vi "Search Remote Session.vi"(8 "error in":errorcluster) -> (0 "error out":errorcluster, 1 "Errors per session try":string[](array[string]), 2 "sessions out":string[][](array[string]))   [LabVIEW 2024, in "Session Scanner.lvlib"]
uses:
  Session Scanner.lvlib
  <vilib>/net/SSH/Client/OpenSSH/OpenSSH Client.lvclass
  C:/Program Files (x86)/National Instruments/LabVIEW 2024/vi.lib/net/SSH/Client/Generic/Generic Client.lvclass
  <vilib>/net/SSH/Client/Generic/Generic Client.lvclass/Generic Client.ctl
  <vilib>/net/SSH/Client/Generic/Write trust on first use.vi
  Support/General Type Defs/Global Data.vi
  <vilib>/net/SSH/NI_SSH.lvlib
  Support/General Type Defs/General Type Defs.lvlib
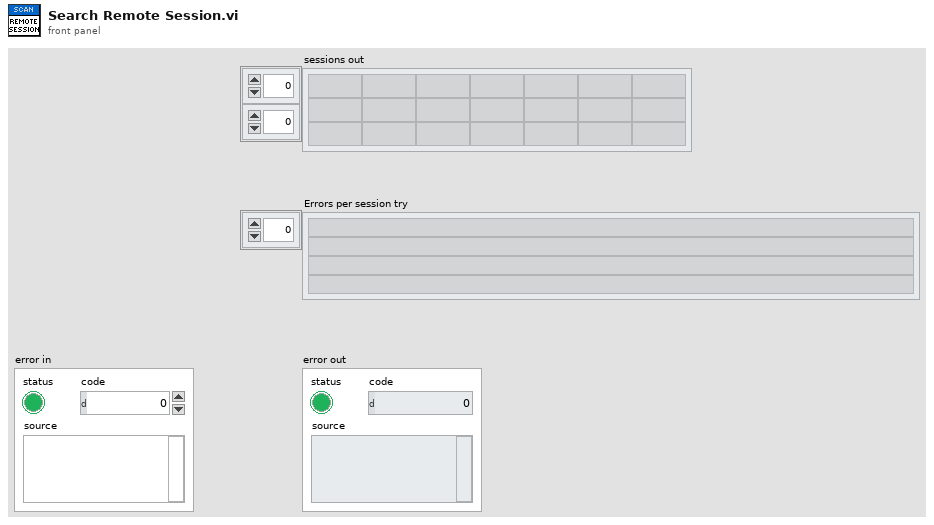
[diagram p1: front panel]
types:
  T1 = typedef "General Type Defs.lvlib/Device Data.ctl" = cluster{"OS":T2, "User":string, "Password":string, "Hostname":string, "IP Address":string}
  T2 = typedef "General Type Defs.lvlib/Device OS.ctl" = enum16{"Windows", "Linux"}
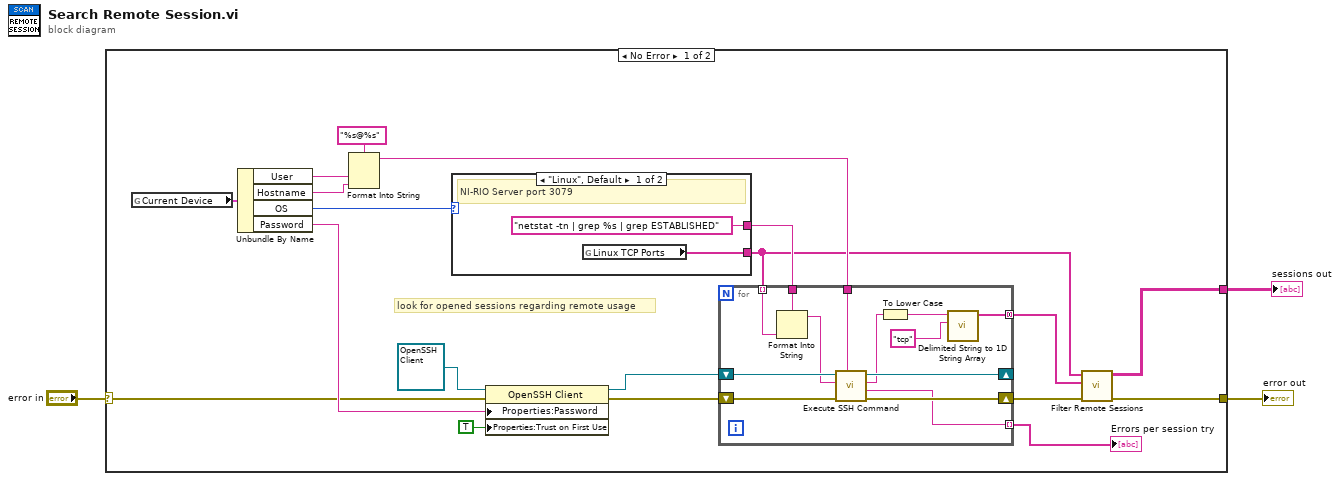
[diagram p0: block diagram]
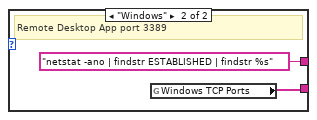
[diagram p2: hidden frame]
diagram:
  n1 = case shown="No Error" "error in" {
    selector: "error in" -> [w14 w40]
    tunnel: [w4 w40] -> w2
    tunnel: [w7 _] -> w1
    frame No Error {
      # "look for opened sessions regarding remote usage"
      n2 = global read "Global Data.vi" "Current Device"() -> (w6:T1)
      n3 = Unbundle By Name(w6) -> ("User"=w17:string, "Hostname"=w16:string, "OS"=w11:T2, "Password"=w15:string)
      n4 = Format Into String(format string="%s@%s", w17, w16) -> (resulting string=w13:string)  [unwired: 2 in, 1 out]
      n5 = case shown="\"Linux\", Default" w11 {
        tunnel: ["netstat -tn | grep %s | grep ESTABLISHED" ("command line") "netstat -ano | findstr ESTABLISHED | findstr %s" ("command line")] -> w12
        tunnel: [w23 w25] -> w8
        frame "Linux", Default {
          # "NI-RIO Server port 3079"
          n6 = global read "Global Data.vi" "Linux TCP Ports"() -> (w23:string[])
        }
        frame "Windows" {
          # "Remote Desktop App port 3389"
          n7 = global read "Global Data.vi" "Windows TCP Ports"() -> (w25:string[])
        }
      }
      n8 = property class="OpenSSH Client"(reference=refnum<class "OpenSSH Client.lvclass"> refnum ("NI_SSH.lvlib:OpenSSH Client"), error in=w14, "Properties:Password"=w15, "Properties:Trust on First Use"=TRUE ("Trust on First Use")) -> (reference out=w19:refnum<class "OpenSSH Client.lvclass">, error out=w20:errorcluster)
      n9 = for {
        tunnel: w13 -> [w36]
        shift-right: [w39] -> w5
        shift-left: w20 -> [w38]
        shift-right: [w35] -> _
        shift-left: w19 -> [w37]
        tunnel: w12 -> [w34]
        tunnel: [w31] -> w9 mode=concatenating
        tunnel: w8 -> [w29] mode=indexing
        tunnel: [w28] -> w10 mode=indexing
        n10 = Format Into String(format string=w34, w29) -> (resulting string=w33:string)  [unwired: 2 in, 1 out]
        n11 = call <vilib>:"Execute SSH Command.vi"("user@host"=w36, "error in (no error)"=w38, "command line"=w33, "session in"=w37) -> ("error out"=w39:errorcluster, "standard error"=w28:string, "standard output"=w32:string, "session out"=w35:refnum<class "OpenSSH Client.lvclass">)  [unwired: 3 in, 1 out]
        n12 = To Lower Case(string=w32) -> (all lower case string=w27:string)
        n13 = call <vilib>:"Delimited String to 1D String Array.vi"("delimiter"="tcp", "delimited string"=w27) -> ("string array"=w31:string[])  [unwired: 9 in]
      }
      "Errors per session try" <- w10
      n14 = call "Filter Remote Sessions.vi"("error in"=w5, "Detected Sessions"=w9, "Windows TCP Ports"=w8) -> ("error out"=w4:errorcluster, "Filtered Remote Sessions"=w7:string[][])  [unwired: 7 in]
    }
    frame Error {
    }
  }
  "error out" <- w2
  "sessions out" <- w1
